vi "Write right SR.vi"(5 "right SR":refnum<class "RightShiftRegister.lvclass">, 9 "ShiftRegister in":refnum<class "ShiftRegister.lvclass">) -> (3 "ShiftRegister out":refnum<class "ShiftRegister.lvclass">)   [LabVIEW 2014, in "ShiftRegister.lvclass"]
uses:
  ShiftRegister.lvclass
  RightShiftRegister/RightShiftRegister.lvclass
  ShiftRegister.lvclass/ShiftRegister.ctl
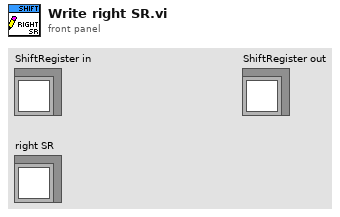
[diagram p1: front panel]
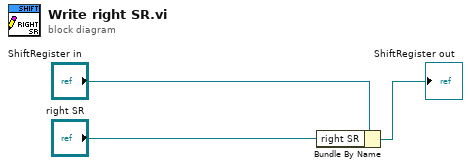
[diagram p0: block diagram]
diagram:
  n1 = Bundle By Name(cluster="ShiftRegister in", "right SR"="right SR") -> (→"ShiftRegister out":refnum<class "ShiftRegister.lvclass">)
